vi "Plot scale range change.vi"(7 "Loop data in":T2={"TitleCollapse"=refnum, "MouseDownState"=enum."Idle", "RightClickCache"={"Mod"={"Ctrl"=FALSE, "Shift"=FALSE}, "CoordsStart"={"Horizontal"=0, "Vertical"=0}, "CoordsEnd"={"Horizontal"=0, "Vertical"=0}, "PlotAreaBounds"={"Left"=10, "Top"=10, "Right"=0, "Bottom"=0}, "slice"=[]}, "ZoomCache"={"SuppressedPlots"=[], "LeftAxis"={"NeedsRevert?"=FALSE, "Scale Fit"=0, "Range"={"Minimum"=0.0, "Maximum"=0.0, "Increment"=0.0, "Minor Increment"=0.0, "Start"=0.0}}, "RightAxis"={"NeedsRevert?"=FALSE, "Scale Fit"=0, "Range"={"Minimum"=0.0, "Maximum"=0.0, "Increment"=0.0, "Minor Increment"=0.0, "Start"=0.0}}, "Mod"={"Shift"=FALSE}}, "UpdateTime"=0.0, "keyboard"=refnum, "visible?"=FALSE}, 8 "error in (no error)":errorcluster, 9 "NewRange":T1, 10 "ScaleRef":refnum<vi>, 11 "Refs":T12) -> (0 "error out":errorcluster, 5 "Loop data out":T2={"TitleCollapse"=refnum, "MouseDownState"=enum."Idle", "RightClickCache"={"Mod"={"Ctrl"=FALSE, "Shift"=FALSE}, "CoordsStart"={"Horizontal"=0, "Vertical"=0}, "CoordsEnd"={"Horizontal"=0, "Vertical"=0}, "PlotAreaBounds"={"Left"=10, "Top"=10, "Right"=0, "Bottom"=0}, "slice"=[]}, "ZoomCache"={"SuppressedPlots"=[], "LeftAxis"={"NeedsRevert?"=FALSE, "Scale Fit"=0, "Range"={"Minimum"=0.0, "Maximum"=0.0, "Increment"=0.0, "Minor Increment"=0.0, "Start"=0.0}}, "RightAxis"={"NeedsRevert?"=FALSE, "Scale Fit"=0, "Range"={"Minimum"=0.0, "Maximum"=0.0, "Increment"=0.0, "Minor Increment"=0.0, "Start"=0.0}}, "Mod"={"Shift"=FALSE}}, "UpdateTime"=0.0, "keyboard"=refnum, "visible?"=FALSE})   [LabVIEW 2021, in "RocketPlot.lvlib"]
uses:
  RocketPlot.lvlib
  TypeDefs/Plot UI references.ctl
  Classes/RocketPlotHandle/RocketPlotHandle.lvclass
  <userlib>/bjustice/TipStripOOPanel/Classes/TipPanelHandle/TipPanelHandle.lvclass
  TypeDefs/Plot top row.ctl
  TypeDefs/plot while loop data.ctl
  CollapsePanel/CollapsePanel.lvclass
  TypeDefs/MouseDownState.ctl
  TypeDefs/RightClickCache.ctl
  TypeDefs/RightClickCache PlatMod.ctl
  <vilib>/Utility/miscctls.llb/LVPoint32TypeDef.ctl
  <vilib>/Utility/miscctls.llb/LVRectTypeDef.ctl
  TypeDefs/Slice average.ctl
  TypeDefs/ZoomCache.ctl
  TypeDefs/RangeCache.ctl
  <vilib>/Utility/miscctls.llb/LVRangeTypeDef.ctl
  TypeDefs/ZoomCache PlatMod.ctl
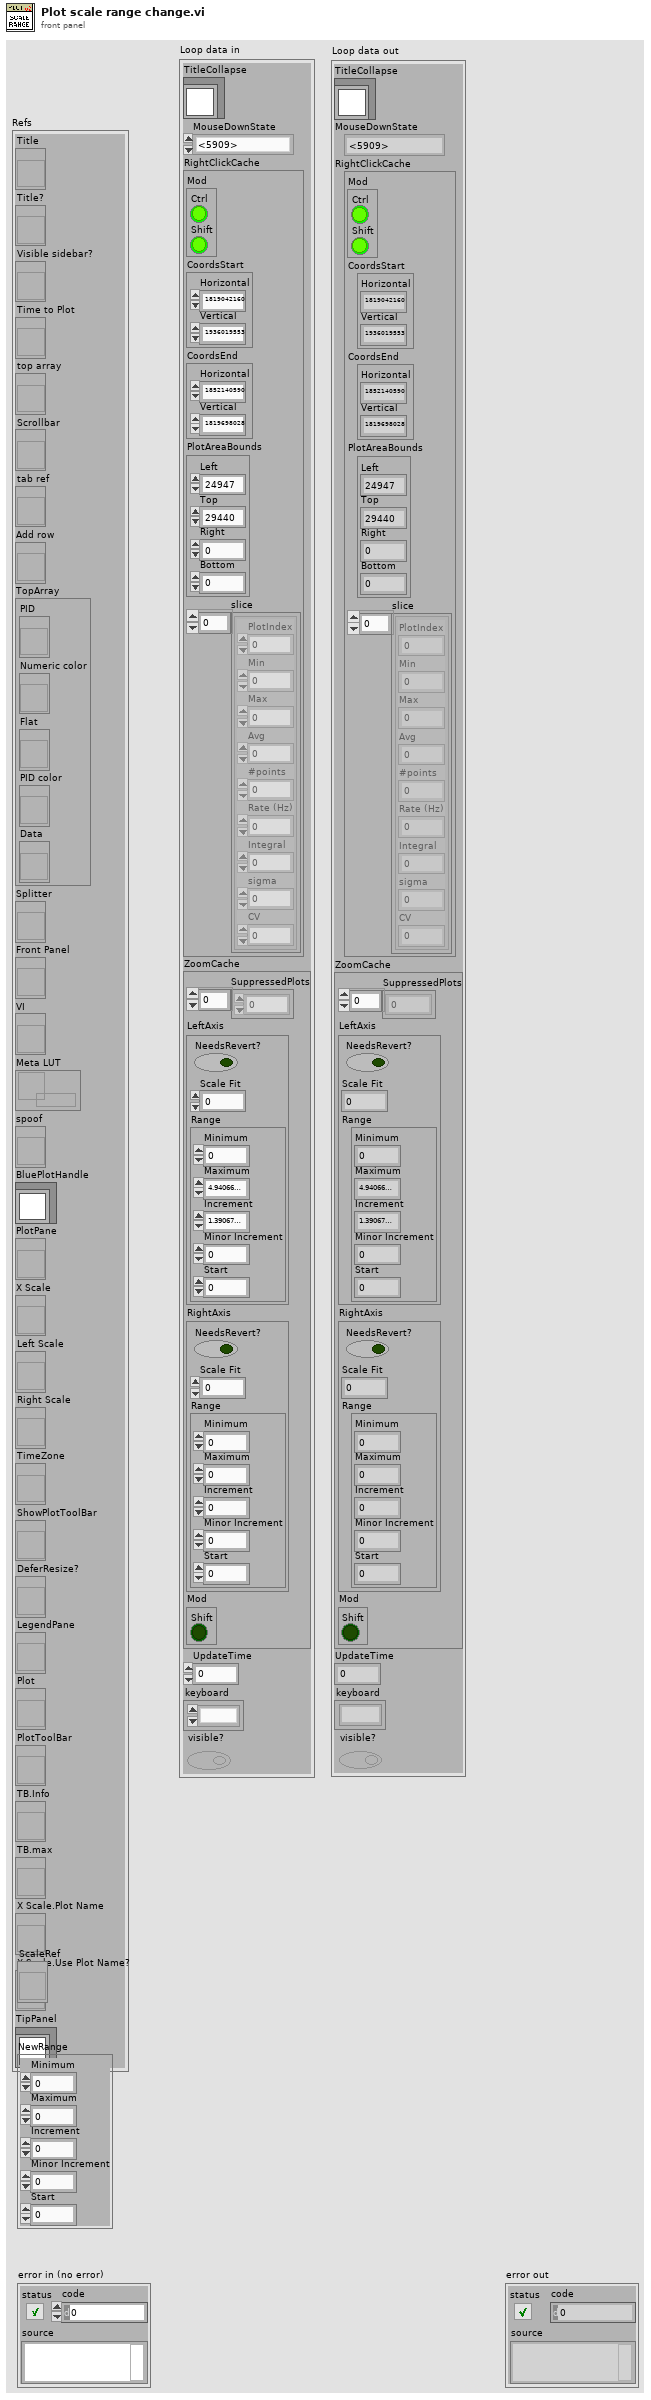
[diagram p1: front panel]
types:
  T1 = typedef "LVRangeTypeDef.ctl" = cluster{"Minimum":dbl, "Maximum":dbl, "Increment":dbl, "Minor Increment":dbl, "Start":dbl}
  T2 = typedef "RocketPlot.lvlib/plot while loop data.ctl" = cluster{"TitleCollapse":refnum<class "CollapsePanel.lvclass">, "MouseDownState":T3, "RightClickCache":T4, "ZoomCache":T9, "UpdateTime":dbl, "keyboard":refnum<k1>, "visible?":bool}
  T3 = typedef "RocketPlot.lvlib/MouseDownState.ctl" = enum16{"Idle", "Pan", "Zoom", "Zoom-Post", "RightClick"}
  T4 = typedef "RocketPlot.lvlib/RightClickCache.ctl" = cluster{"Mod":T5, "CoordsStart":T6, "CoordsEnd":T6, "PlotAreaBounds":T7, "slice":T8[]}
  T5 = typedef "RocketPlot.lvlib/RightClickCache PlatMod.ctl" = cluster{"Ctrl":bool, "Shift":bool}
  T6 = typedef "LVPoint32TypeDef.ctl" = cluster{"Horizontal":i32, "Vertical":i32}
  T7 = typedef "LVRectTypeDef.ctl" = cluster{"Left":i16, "Top":i16, "Right":i16, "Bottom":i16}
  T8 = typedef "RocketPlot.lvlib/Slice average.ctl" = cluster{"PlotIndex":i32, "Min":dbl, "Max":dbl, "Avg":dbl, "#points":u32, "Rate (Hz)":dbl, "Integral":dbl, "sigma":dbl, "CV":dbl}
  T9 = typedef "RocketPlot.lvlib/ZoomCache.ctl" = cluster{"SuppressedPlots":i32[], "LeftAxis":T10, "RightAxis":T10, "Mod":T11}
  T10 = typedef "RocketPlot.lvlib/RangeCache.ctl" = cluster{"NeedsRevert?":bool, "Scale Fit":u8, "Range":T1}
  T11 = typedef "RocketPlot.lvlib/ZoomCache PlatMod.ctl" = cluster{"Shift":bool}
  T12 = typedef "RocketPlot.lvlib/Plot UI references.ctl" = cluster{"Title":refnum<vi>, "Title?":refnum<vi>, "Visible sidebar?":refnum<vi>, "Time to Plot":refnum<vi>, "top array":refnum<vi>, "Scrollbar":refnum<vi>, "tab ref":refnum<vi>, "Add row":refnum<vi>, "TopArray":cluster{"PID":refnum<vi>, "Numeric color":refnum<vi>, "Flat":refnum<vi>, "PID color":refnum<vi>, "Data":refnum<vi>}, "Splitter":refnum<vi>, "Front Panel":refnum<vi>, "VI":refnum<vi>, "Meta LUT":refnum<data-value>, "spoof":refnum<vi>, "BluePlotHandle":refnum<class "RocketPlotHandle.lvclass">, "PlotPane":refnum<vi>, "X Scale":refnum<vi>, "Left Scale":refnum<vi>, "Right Scale":refnum<vi>, "TimeZone":refnum<vi>, "ShowPlotToolBar":refnum<vi>, "DeferResize?":refnum<vi>, "LegendPane":refnum<vi>, "Plot":refnum<vi>, "PlotToolBar":refnum<vi>, "TB.Info":refnum<vi>, "TB.max":refnum<vi>, "X Scale.Plot Name":refnum<vi>, "X Scale.Use Plot Name?":refnum<vi>, "TipPanel":refnum<class "TipPanelHandle.lvclass">}
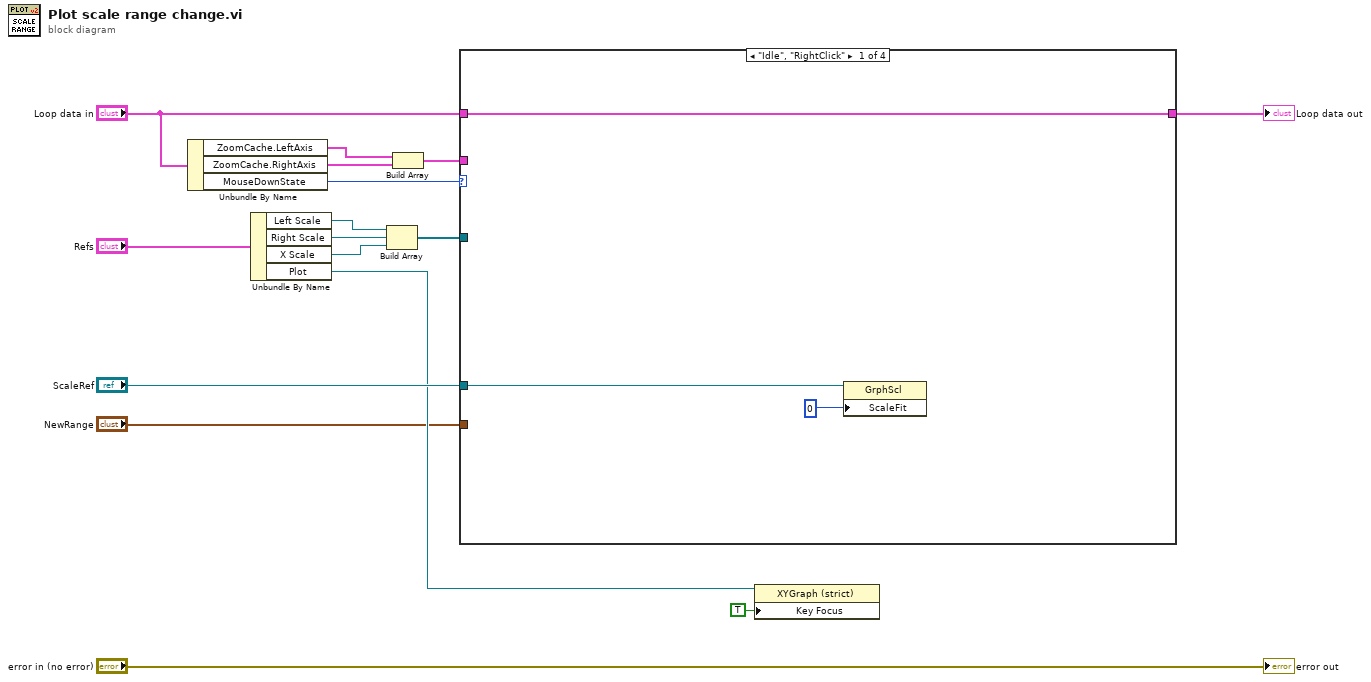
[diagram p0: block diagram]
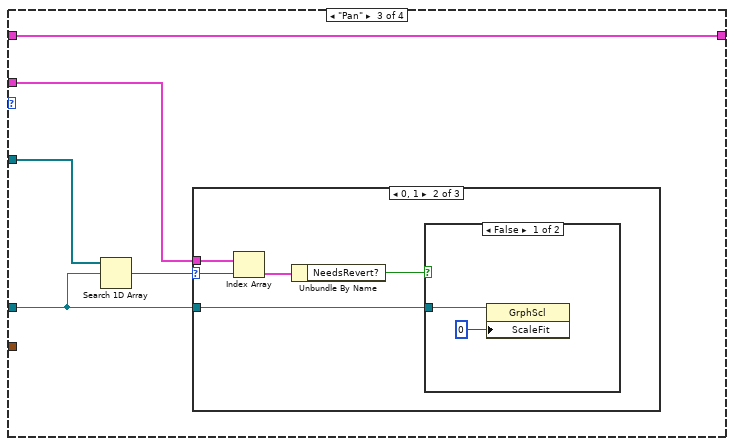
[diagram p3: hidden frame]
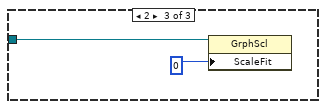
[diagram p6: hidden frame]
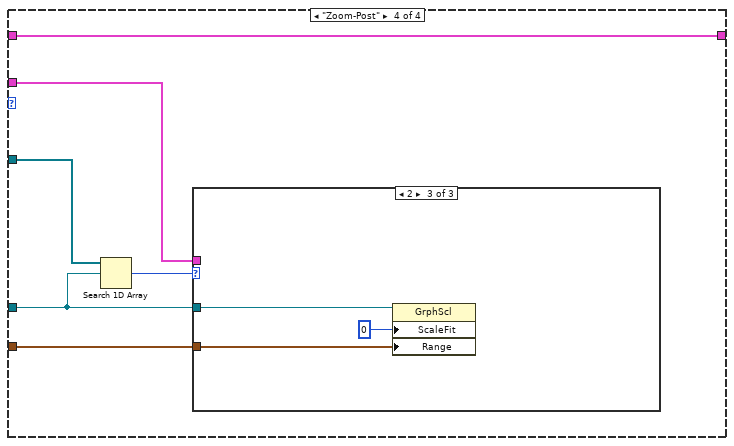
[diagram p7: hidden frame]
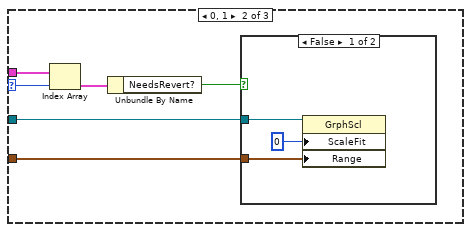
[diagram p9: hidden frame]
diagram:
  n1 = Unbundle By Name("Loop data in") -> ("ZoomCache.LeftAxis"=w13:T10, "ZoomCache.RightAxis"=w12:T10, "MouseDownState"=w5:T3)
  n2 = Unbundle By Name("Refs") -> ("Left Scale"=w15:refnum<vi>, "Right Scale"=w14:refnum<vi>, "X Scale"=w7:refnum<vi>, "Plot"=w8:refnum<vi>)
  n3 = Build Array(w15, w14, w7) -> (w11:refnum<vi>[])
  n4 = Build Array(w13, w12) -> (w9:T10[])
  n5 = case shown="\"Idle\", \"RightClick\"" w5 {
    tunnel: w11 -> [_ _ w25 w40]
    tunnel: "ScaleRef" -> [w19 _ w24 w39]
    tunnel: w9 -> [_ _ w22 w37]
    tunnel: "NewRange" -> [_ _ _ w35]
    tunnel: "Loop data in" -> [w17 w20 w21 w36]
    tunnel: [w17 w20 w21 w36] -> w2
    frame "Idle", "RightClick" {
      n6 = property class="GrphScl"(reference=w19, "ScaleFit"=u8 0 ("Scale Fit")) -> ()  [unwired: 1 in, 2 out]
    }
    frame "Zoom" {
    }
    frame "Pan" {
      n7 = Search 1D Array(1D array=w25, element=w24) -> (index of element=w23:i32)  [unwired: 1 in]
      n8 = case shown="0, 1" w23 {
        selector: w23 -> [_ w28 _]
        tunnel: w24 -> [_ w30 w33]
        tunnel: w22 -> [_ w29 _]
        frame -1, Default {
        }
        frame 0, 1 {
          n9 = Index Array(array=w29, index=w28) -> (element=w27:T10)
          n10 = Unbundle By Name(w27) -> ("NeedsRevert?"=w26:bool)
          n11 = case shown="False" w26 {
            tunnel: w30 -> [w31 _]
            frame False {
              n12 = property class="GrphScl"(reference=w31, "ScaleFit"=u8 0 ("Scale Fit")) -> ()  [unwired: 1 in, 2 out]
            }
            frame True {
            }
          }
        }
        frame 2 {
          n13 = property class="GrphScl"(reference=w33, "ScaleFit"=u8 0 ("Scale Fit")) -> ()  [unwired: 1 in, 2 out]
        }
      }
    }
    frame "Zoom-Post" {
      n14 = Search 1D Array(1D array=w40, element=w39) -> (index of element=w38:i32)  [unwired: 1 in]
      n15 = case shown="2" w38 {
        selector: w38 -> [_ w44 _]
        tunnel: w39 -> [_ w46 w51]
        tunnel: w37 -> [_ w45 _]
        tunnel: w35 -> [_ w41 w50]
        frame -1, Default {
        }
        frame 0, 1 {
          n16 = Index Array(array=w45, index=w44) -> (element=w43:T10)
          n17 = Unbundle By Name(w43) -> ("NeedsRevert?"=w42:bool)
          n18 = case shown="False" w42 {
            tunnel: w46 -> [w48 _]
            tunnel: w41 -> [w47 _]
            frame False {
              n19 = property class="GrphScl"(reference=w48, "ScaleFit"=u8 0 ("Scale Fit"), "Range"=w47) -> ()  [unwired: 1 in, 2 out]
            }
            frame True {
            }
          }
        }
        frame 2 {
          n20 = property class="GrphScl"(reference=w51, "ScaleFit"=u8 0 ("Scale Fit"), "Range"=w50) -> ()  [unwired: 1 in, 2 out]
        }
      }
    }
  }
  "Loop data out" <- w2
  n21 = property class="XYGraph (strict)"(reference=w8, "Key Focus"=TRUE) -> ()  [unwired: 1 in, 2 out]
  "error out" <- "error in (no error)"
